vi "Menu Act open file.vi"(8 "error in (no error)":errorcluster, 11 "LF2R IDE in":refnum<class "Main Panel.lvclass">) -> (0 "error out":errorcluster, 3 "LF2R IDE out":refnum<class "Main Panel.lvclass">)   [LabVIEW 2018, in "Main Panel.lvlib" / "Main Panel.lvclass"]
uses:
  Main Panel.lvclass
  Main Panel.lvclass/Main Panel.ctl
  ScintillaNET/ScintillaNET.lvclass
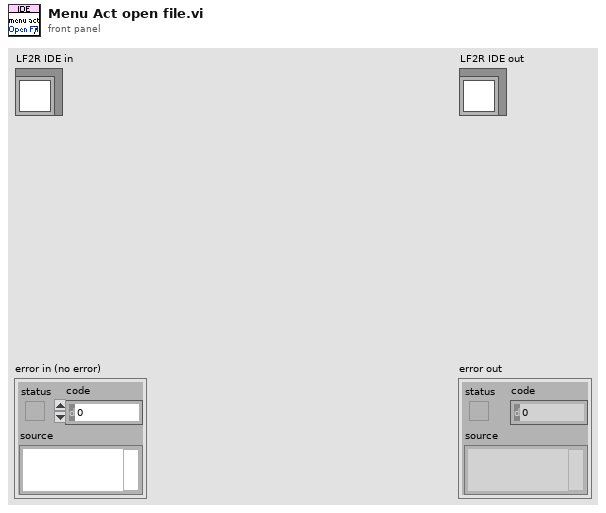
[diagram p1: front panel]
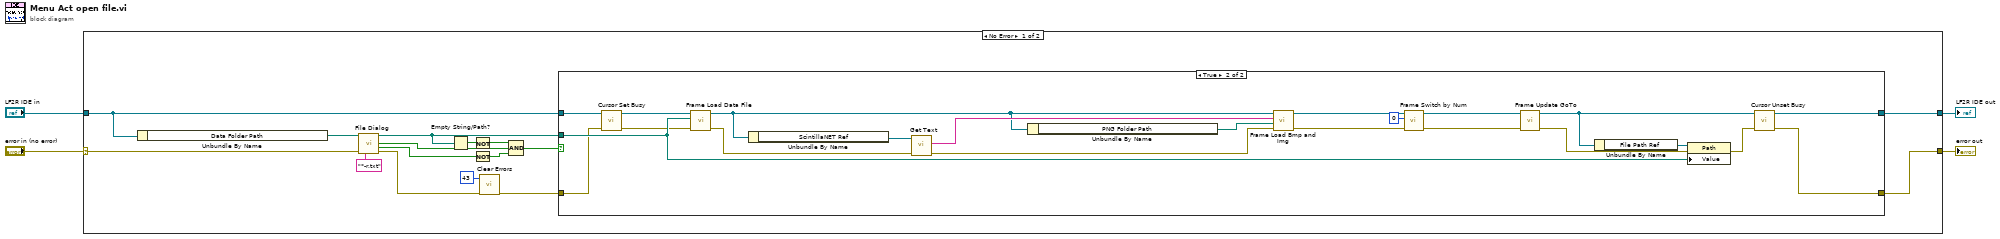
[diagram p0: block diagram]
diagram:
  n1 = case shown="No Error" "error in (no error)" {
    selector: "error in (no error)" -> [w11 w46]
    tunnel: [w19 w46] -> w3
    tunnel: [w20 w45] -> w1
    tunnel: "LF2R IDE in" -> [w9 w45]
    frame No Error {
      n2 = Unbundle By Name(w9) -> ("Data Folder Path"=w8:path)
      n3 = call "File Dialog"("start path"=w8, "error in"=w11, "pattern (all files)"="*-r.txt" ("pattern label")) -> ("selected path"=w12:path, "exists"=w15:bool, "cancelled"=w18:bool, "error out"=w7:errorcluster)  [unwired: 9 in]
      n4 = Empty String/Path?(string/path=w12) -> (empty?=w17:bool)
      n5 = Not(x=w17) -> (.not. x?=w16:bool)
      n6 = Not(x=w18) -> (.not. x?=w14:bool)
      n7 = call <vilib>:"Clear Errors.vi"("error in (no error)"=w7, "specific error code to clear (0: all)"=43) -> ("error out"=w6:errorcluster)  [unwired: 4 in, 1 out]
      n8 = Compound Arithmetic op=AND(w16, w15, w14) -> (w13:bool)
      n9 = case shown="True" w13 {
        tunnel: [w22 w33] -> w20
        tunnel: [w21 w31] -> w19
        tunnel: w9 -> [w22 w38]
        tunnel: w12 -> [_ w44]
        tunnel: w6 -> [w21 w35]
        frame False {
        }
        frame True {
          n10 = call "Cursor Set Busy.vi"("error in (no error)"=w35, "LF2R IDE in"=w38) -> ("error out"=w36:errorcluster, "LF2R IDE out"=w37:refnum<class "Main Panel.lvclass">)  [unwired: 8 in]
          n11 = call "Frame Load Data File.vi"("error in (no error)"=w36, "File Path"=w44, "IDE simple in"=w37) -> ("error out"=w40:errorcluster, "IDE simple out"=w24:refnum<class "Main Panel.lvclass">)  [unwired: 7 in]
          n12 = Unbundle By Name(w24) -> ("ScintillaNET Ref"=w41:refnum<class "ScintillaNET.lvclass">)
          n13 = call "Get Text.vi"("error in (no error)"=w40, "ScintillaNET in"=w41) -> ("error out"=w25:errorcluster, "Text"=w39:string)  [unwired: 7 in, 1 out]
          n14 = Unbundle By Name(w24) -> ("PNG Folder Path"=w23:path)
          n15 = call "Frame Load Bmp and Img.vi"("error in (no error)"=w25, "PNG Path"=w23, "File String"=w39, "LF2R IDE in"=w24) -> ("error out"=w29:errorcluster, "LF2R IDE out"=w30:refnum<class "Main Panel.lvclass">)  [unwired: 6 in]
          n16 = call "Frame Switch by Num.vi"("error in (no error)"=w29, "Frame Num"=u32 0, "LF2R IDE in"=w30) -> ("error out"=w27:errorcluster, "LF2R IDE out"=w28:refnum<class "Main Panel.lvclass">)  [unwired: 7 in]
          n17 = call "Frame Update GoTo.vi"("error in (no error)"=w27, "LF2R IDE in"=w28) -> ("error out"=w43:errorcluster, "LF2R IDE out"=w34:refnum<class "Main Panel.lvclass">)  [unwired: 8 in]
          n18 = Unbundle By Name(w34) -> ("File Path Ref"=w42:refnum<vi>)
          n19 = property class="Path"(reference=w42, error in=w43, "Value"=w44) -> (error out=w32:errorcluster)  [unwired: 1 out]
          n20 = call "Cursor Unset Busy.vi"("error in (no error)"=w32, "LF2R IDE in"=w34) -> ("error out"=w31:errorcluster, "LF2R IDE out"=w33:refnum<class "Main Panel.lvclass">)  [unwired: 8 in]
        }
      }
    }
    frame Error {
    }
  }
  "error out" <- w3
  "LF2R IDE out" <- w1
